vi "Node LUT.vi"(6 "Command":T2, 8 "error in":errorcluster, 9 "node ref":T1, 10 "UID":string) -> (0 "error out":errorcluster, 1 "node ref":T1, 2 "node refs":T1[](array[typedef]), 3 "UIDs":string[](array[string]))   [LabVIEW 2015, in "Node LUT.lvlib"]
uses:
  Node LUT.lvlib
  <vilib>/NI/Configuration Framework/Node/NISE_CEF_Node.lvclass
  Command.ctl
  <vilib>/NI/Configuration Framework/Node/NodeRef.ctl
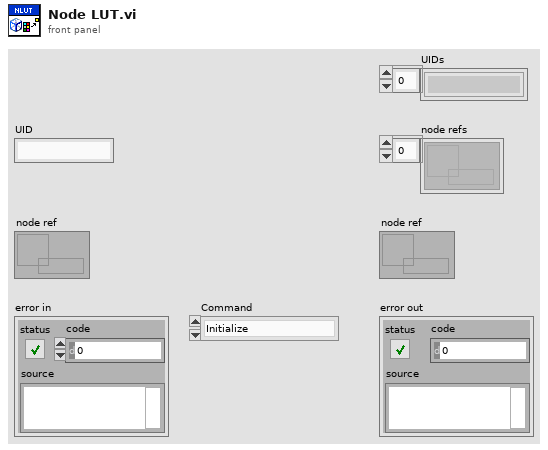
[diagram p1: front panel]
types:
  T1 = typedef "NISE_CEF_Node.lvclass/NodeRef.ctl" = refnum<data-value>
  T2 = typedef "Node LUT.lvlib/Command.ctl" = enum16{"Initialize", "Add Node", "Remove Node", "Node Ref from UID", "List Nodes"}
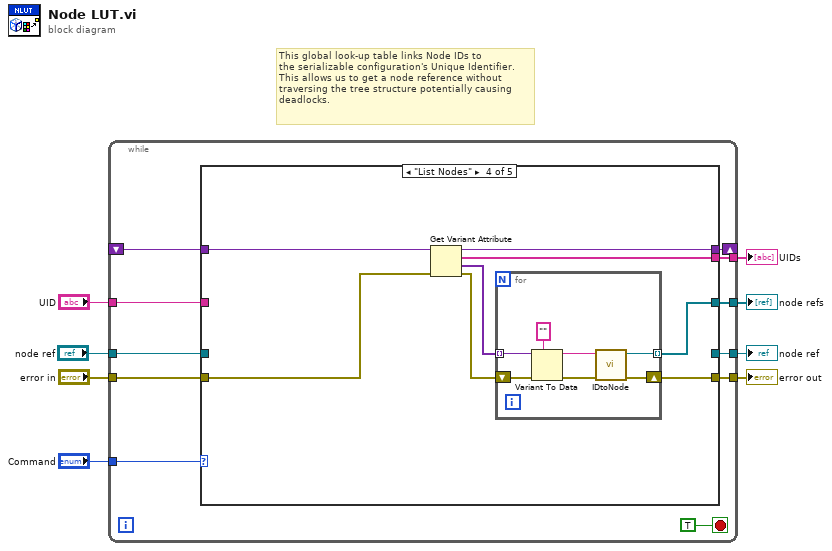
[diagram p0: block diagram]
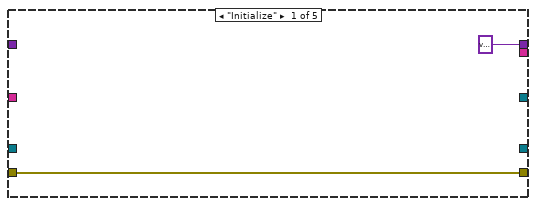
[diagram p2: hidden frame]
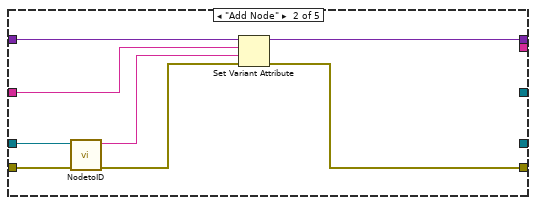
[diagram p3: hidden frame]
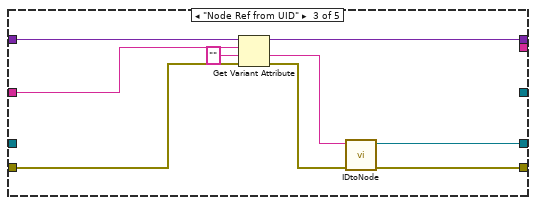
[diagram p4: hidden frame]
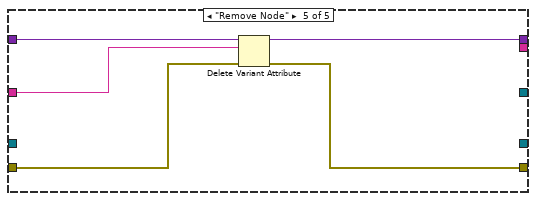
[diagram p5: hidden frame]
diagram:
  # "This global look-up table links Node IDs to\nthe serializable configuration's Unique Identifier.\nThis allows us to get a node reference without\ntraversing the tree structure potentially causing\ndeadlocks."
  n1 = while {
    tunnel: "Command" -> [w18]
    shift-right: [w17] -> _
    shift-left: _ -> [w16]
    tunnel: [w15] -> w7
    tunnel: "error in" -> [w14]
    tunnel: "UID" -> [w13]
    tunnel: "node ref" -> [w12]
    tunnel: [w11] -> w3
    tunnel: [w10] -> w2
    tunnel: [w9] -> w1
    stop <- TRUE stop-if-true
    n2 = case shown="\"List Nodes\"" w18 {
      tunnel: [variant w28 w37 w45 w58] -> w17
      tunnel: w16 -> [_ w29 w38 w46 w54]
      tunnel: [w20 w27 w32 w42 w57] -> w15
      tunnel: w14 -> [w20 w25 w35 w44 w56]
      tunnel: w13 -> [_ w26 w36 _ w55]
      tunnel: w12 -> [_ w22 _ _ _]
      tunnel: [_ _ _ w40 _] -> w11
      tunnel: [_ _ _ w39 _] -> w10
      tunnel: [_ _ w30 _ _] -> w9
      frame "Initialize" {
      }
      frame "Add Node" {
        n3 = call <vilib>:"NodetoID.vi"("error in"=w25, "node ref"=w22) -> ("error out"=w24:errorcluster, "ID"=w23:string)  [unwired: 8 in]
        n4 = Set Variant Attribute(Variant=w29, name=w26, value=w23, error in=w24) -> (Variant out=w28:variant, error out=w27:errorcluster)  [unwired: 1 out]
      }
      frame "Node Ref from UID" {
        n5 = Get Variant Attribute(Variant=w38, name=w36, default value (empty Variant)="", error in=w35) -> (duplicate Variant=w37:variant, value=w31:string, error out=w33:errorcluster)  [unwired: 1 out]
        n6 = call <vilib>:"IDtoNode.vi"("error in"=w33, "ID"=w31) -> ("error out"=w32:errorcluster, "node ref"=w30:T1)  [unwired: 7 in, 1 out]
      }
      frame "List Nodes" {
        n7 = Get Variant Attribute(Variant=w46, error in=w44) -> (duplicate Variant=w45:variant, names=w39:string[], values=w43:variant[], error out=w41:errorcluster)  [unwired: 2 in]
        n8 = for {
          tunnel: w43 -> [w53] mode=indexing
          shift-right: [w48] -> w42
          shift-left: w41 -> [w52]
          tunnel: [w47] -> w40 mode=indexing
          n9 = Variant To Data(error in=w52, type="", Variant=w53) -> (data=w50:string, error out=w49:errorcluster)
          n10 = call <vilib>:"IDtoNode.vi"("error in"=w49, "ID"=w50) -> ("error out"=w48:errorcluster, "node ref"=w47:T1)  [unwired: 7 in, 1 out]
        }
      }
      frame "Remove Node" {
        n11 = Delete Variant Attribute(4:w56, 6:w55, 7:w54) -> (0:w57:errorcluster, 3:w58:variant)  [unwired: 1 out]
      }
    }
  }
  "error out" <- w7
  "node refs" <- w3
  "UIDs" <- w2
  "node ref" <- w1
